vi "XIPIN_Distributed_Memory_Generator_8_0.vi"   [LabVIEW 2017]
doc: "The LogiCORE Xilinx Distributed Memory Generator creates area and performance optimized ROM blocks, single, dual and simple dual port distributed memories for Xilinx FPGAs. The core supersedes the previously released LogiCORE Distributed Memory core. Use this core in all new designs for supported families wherever a distributed memory is required.\n------------------------------------\n<b>Need License</b> : No"
uses:
  <vilib>/rvi/XilinxIP/XIPIN_XNode/niFpgaXIPIN.xnode
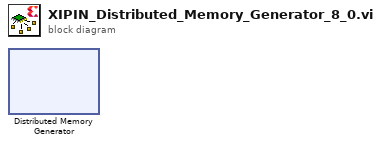
[diagram p0: block diagram]
diagram:
  n1 = xnode ("Distributed Memory Generator")() -> ()
